vi "check timing board (SubVI).vi"(8 "errIN":errorcluster, 10 "ActiveDev":tag="LightScreens", 11 "measSrc_ref":refnum<vi>) -> (0 "error out":errorcluster, 3 "deviceID":string)   [LabVIEW 2015]
uses:
  DataSource.ctl
  <resource>/objmgr/daqmx.rc
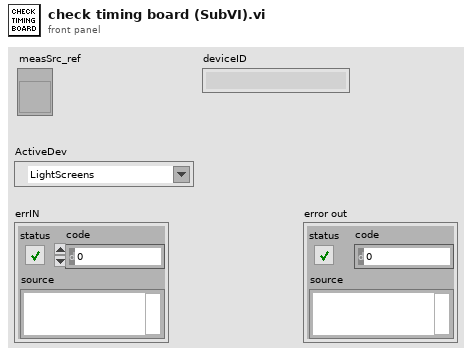
[diagram p1: front panel]
types:
  T1 = typedef "DataSource.ctl" = enum16{"Simulated", "Radar", "Screens"}
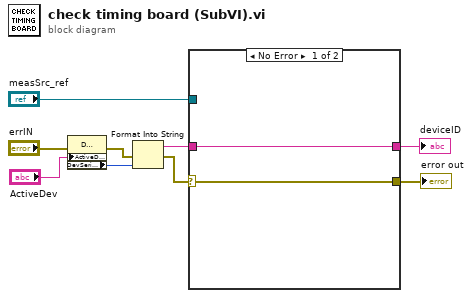
[diagram p0: block diagram]
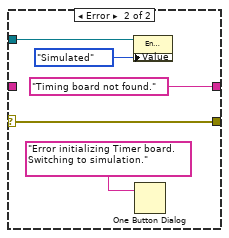
[diagram p2: hidden frame]
diagram:
  n1 = property class="DAQmx Device"(error in="errIN", "ActiveDev"="ActiveDev") -> (error out=w8:errorcluster, "DevSerialNum"=w6:u32)  [unwired: 1 in, 1 out]
  n2 = Format Into String(error in=w8, w6) -> (resulting string=w7:string, error out=w9:errorcluster)  [unwired: 2 in]
  n3 = case shown="No Error" w9 {
    selector: w9 -> [w10 w12]
    tunnel: w7 -> [w11 _]
    tunnel: [w11 "Timing board not found." ("information string")] -> w2
    tunnel: [w10 w12] -> w3
    tunnel: "measSrc_ref" -> [_ w13]
    frame No Error {
    }
    frame Error {
      n4 = property class="Enum (strict)"(reference=w13, "Value"=DataSource."Simulated" ("MeasSrc")) -> ()  [unwired: 1 in, 2 out]
      n5 = One Button Dialog(message="Error initializing Timer board.  Switching to simulation.") -> ()  [unwired: 2 out]
    }
  }
  "error out" <- w3
  "deviceID" <- w2
